vi "Contour Plot (Filled).vi"() -> ()   [LabVIEW 2011]
uses:
  <vilib>/Heliosphere Research LLC/Advanced Plotting Toolkit/Advanced Plotting Toolkit.lvlib
  <vilib>/Heliosphere Research LLC/Advanced Plotting Toolkit/api_plotting/ContourFilled_Automatic.vi
  <vilib>/Heliosphere Research LLC/Advanced Plotting Toolkit/api_plotting/ContourFilled_Manual.vi
  <vilib>/Heliosphere Research LLC/Advanced Plotting Toolkit/properties/Colormap_Map.ctl
  <vilib>/Heliosphere Research LLC/Advanced Plotting Toolkit/properties/Colormap_Scaling.ctl
  <vilib>/Heliosphere Research LLC/Advanced Plotting Toolkit/properties/Colormap.ctl
  <vilib>/Heliosphere Research LLC/Advanced Plotting Toolkit/properties/Display.ctl
  <vilib>/Heliosphere Research LLC/Advanced Plotting Toolkit/api_plotting/ContourFilledProperties.ctl
panel:
  in  "Colormap":T1=enum."Hot and Cold"
  in  "Auto Contour":bool=TRUE
  in  "Manual Contours":dbl[](array[numeric])=[-0.75, 0.0, 0.125, 1.0]
  in  "Number of Automatic Contours":i32=20
  out "Filled Contour Plot":picture
  # "Filled Contour Plot"
  # "This VI demonstrates an alternative form of contour plot, in\ncontast to Contour.vi.  Here, data is visualized as colored\nbands between contours.\n\nLike Contour.vi, provide a 2D dataset to visualize, and\nspecify the desired levels.  ContourFilled.vi is polymorphic,\nand adapts to two data types for the levels: an integer\ngiving the total number of levels (automatic contouring),\nor an array explicitly listing the levels to contour.\n\nLevels are shaded according to a selectable colormap.\nTry changing the colormap in use below.\n\nIf both lines and filled contours are desired, simply call\nboth this VI and Contour.vi on the same plot."
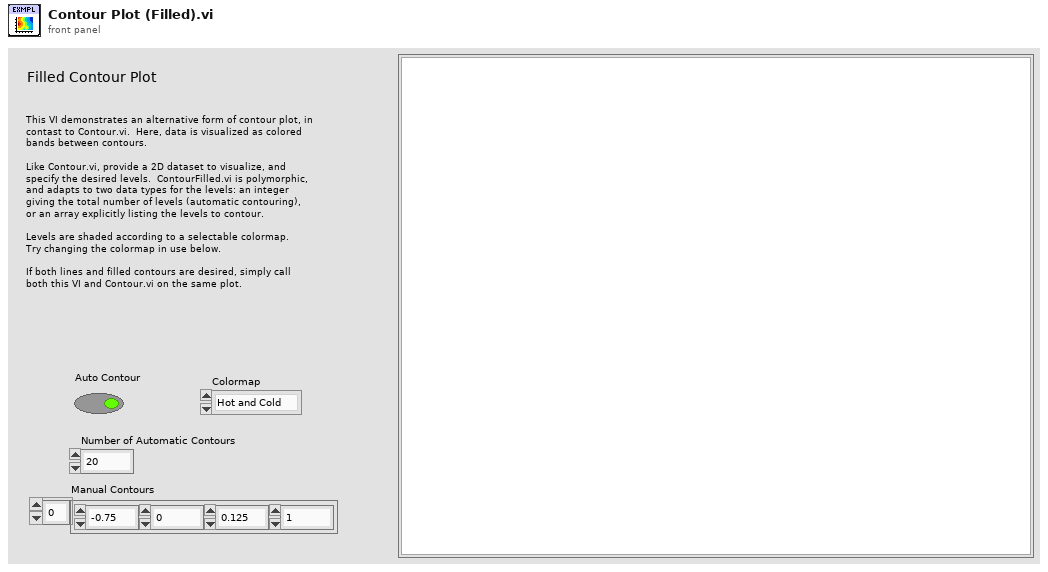
[diagram p1: front panel]
types:
  T1 = typedef "Advanced Plotting Toolkit.lvlib/Colormap_Map.ctl" = enum16{"Automatic", "Rainbow", "Hot and Cold", "White-Black", "White-Blue", "White-Green", "White-Red", "Fire", "Water", "Earth", "Air", "Pastel", "Banded", "Stepped"}
  T2 = typedef "Advanced Plotting Toolkit.lvlib/ContourFilledProperties.ctl" = cluster{"Colormap":T3, "Display":T5}
  T3 = typedef "Advanced Plotting Toolkit.lvlib/Colormap.ctl" = cluster{"Map":T1, "Value Min":dbl, "Value Max":dbl, "Scaling":T4, "Reverse":bool}
  T4 = typedef "Advanced Plotting Toolkit.lvlib/Colormap_Scaling.ctl" = enum16{"Default"}
  T5 = typedef "Advanced Plotting Toolkit.lvlib/Display.ctl" = cluster{"Alpha":dbl, "Z Order":dbl}
  T6 = typedef "Advanced Plotting Toolkit.lvlib/PlotID.ctl" = i32
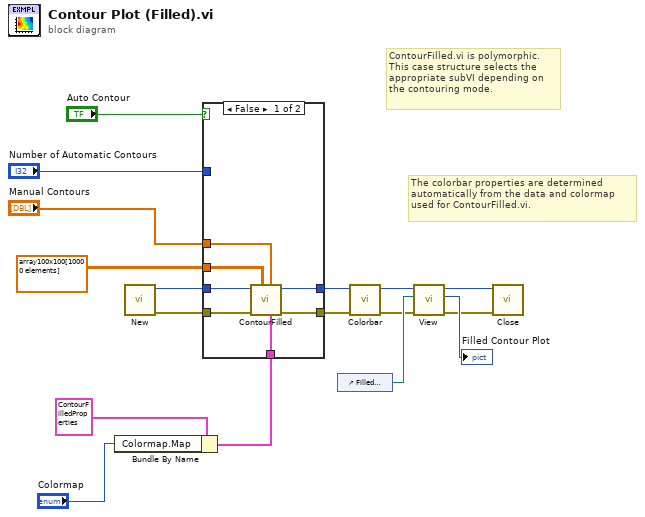
[diagram p0: block diagram]
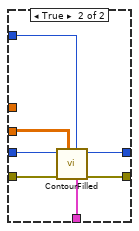
[diagram p2: hidden frame]
diagram:
  # "The colorbar properties are determined\nautomatically from the data and colormap\nused for ContourFilled.vi."
  # "ContourFilled.vi is polymorphic.\nThis case structure selects the\nappropriate subVI depending on\nthe contouring mode."
  n1 = Bundle By Name(cluster=T2 {"Colormap"={"Map"=enum."Automatic", "Value Min"=nan, "Value Max"=nan, "Scaling"=enum."Default", "Reverse"=FALSE}, "Display"={"Alpha"=nan, "Z Order"=nan}} ("Filled Contour Properties"), "Colormap.Map"="Colormap") -> (w9:T2)
  n2 = call <vilib>:"New.vi"() -> ("error out"=w4:errorcluster, "Plot ID"=w5:T6)  [unwired: 10 in]
  n3 = case shown="False" "Auto Contour" {
    tunnel: [w21 w31] -> w7
    tunnel: w5 -> [w22 w30]
    tunnel: sgl[][] array100x100[10000 elements] ("Array") -> [w24 w29]
    tunnel: w9 -> [w23 w28]
    tunnel: "Number of Automatic Contours" -> [_ w27]
    tunnel: "Manual Contours" -> [w20 _]
    tunnel: w4 -> [w19 w26]
    tunnel: [w18 w25] -> w3
    frame False {
      n4 = call-poly <vilib>:"ContourFilled.vi"("Properties"=w23, "Levels"=w20, "Z Data"=w24, "error in (no error)"=w19, "Plot ID"=w22) -> ("error out"=w18:errorcluster, "Plot ID Out"=w21:T6)  [unwired: 5 in]
    }
    frame True {
      n5 = call-poly <vilib>:"ContourFilled.vi"("Properties"=w28, "Levels"=w27, "Z Data"=w29, "error in (no error)"=w26, "Plot ID"=w30) -> ("error out"=w25:errorcluster, "Plot ID Out"=w31:T6)  [unwired: 5 in]
    }
  }
  n6 = control-ref of="Filled Contour Plot"() -> (w17:refnum<vi>)
  n7 = call <vilib>:"Colorbar.vi"("error in (no error)"=w3, "Plot ID"=w7) -> ("error out"=w2:errorcluster, "Plot ID Out"=w6:T6)  [unwired: 8 in]
  n8 = call <vilib>:"View.vi"("error in (no error)"=w2, "Ref for Sizing"=w17, "Plot ID"=w6) -> ("error out"=w1:errorcluster, "Picture"=→"Filled Contour Plot":picture, "Plot ID Out"=w15:T6)  [unwired: 6 in]
  n9 = call <vilib>:"Close.vi"("error in (no error)"=w1, "Plot ID"=w15) -> ()  [unwired: 9 in, 1 out]
